vi "Day4_Statistics.vi"() -> ()   [LabVIEW 2025]
uses:
  <vilib>/Platform/TimedLoop/XDataNode/timing_clust.ctl
  <vilib>/Platform/TimedLoop/XDataNode/nitl_modes.ctl
  <vilib>/Platform/TimedLoop/XDataNode/wakeup.ctl
  <vilib>/Utility/error.llb/Trim Whitespace One-Sided.vi
  <vilib>/Instr/_visa.llb/VISA Configure Serial Port (Instr).vi
  <vilib>/platform/TimedLoop/XDataNode/XDataNode.xnode
  <vilib>/Platform/TimedLoop/XDataNode/XDNodeRunTimeDep.lvlib
  <vilib>/ptbypt/NI_PtbyPt.lvlib
panel:
  out "Max":dbl
  out "Min":dbl
  out "Mean":dbl
  out "Std Dev":dbl
  out "mean":dbl format="%0.2f"
  out "ADC (mv)":dbl
  out "Touch Pin":dbl
  out "Hall Sensor":dbl
  out "Timestamp":dbl
  in  "stop":bool
  # "Day 4: Statistics engine using a custom SubVI. Collects last 20 Touch Pin readings and computes live stats"
  # "Mean PtByPt: continuous running average since session start"
  # "Stats SubVI outputs: computed from a rolling buffer of the last 20 Touch Pin samples."
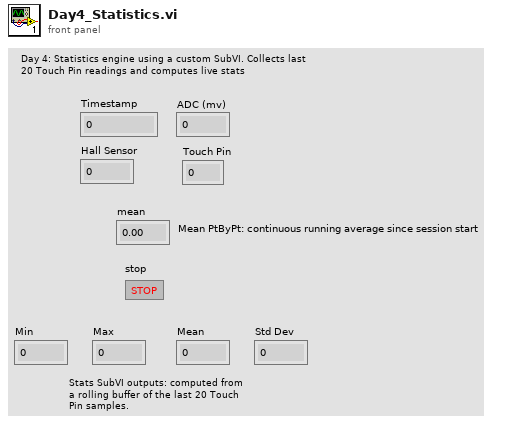
[diagram p1: front panel]
types:
  T1 = typedef "XDNodeRunTimeDep.lvlib/timing_clust.ctl" = cluster{"Expected End [f-1]":u64, "Actual End [f-1]":u64, "Finished Late? [f-1]":bool, "Expected End [i-1]":u64, "Actual End [i-1]":u64, "Finished Late? [i-1]":bool, "Expected Start [i]":u64, "Actual Start [i]":u64, "Expected Start [f]":u64, "Actual Start [f]":u64, "Source Name":string, "Structure Name":string, "Period":i64, "Deadline":i64, "Offset":i64, "Start":i64, "Priority":i32, "Timeout":i32, "Mode":T2, "Wakeup Reason":T3, "Error":errorcluster, "Source Type":string, "Secondary Source Type":string, "Global End Time":u64, "Global Start Time":u64, "Frame Duration":u64, "Iteration Duration":u64, "Assigned CPU":i32, "I/O Scan Engine Mode":u32}
  T2 = typedef "XDNodeRunTimeDep.lvlib/nitl_modes.ctl" = enum32{"No Change", "Process missed periods, maintain original phase", "Discard missed periods, maintain original phase", "Process missed periods, ignore original phase", "Discard missed periods, ignore original phase"}
  T3 = typedef "XDNodeRunTimeDep.lvlib/wakeup.ctl" = enum32{"Normal", "Aborted", "Asynchronous wakeup", "Timing source error", "Timed loop error", "Timeout"}
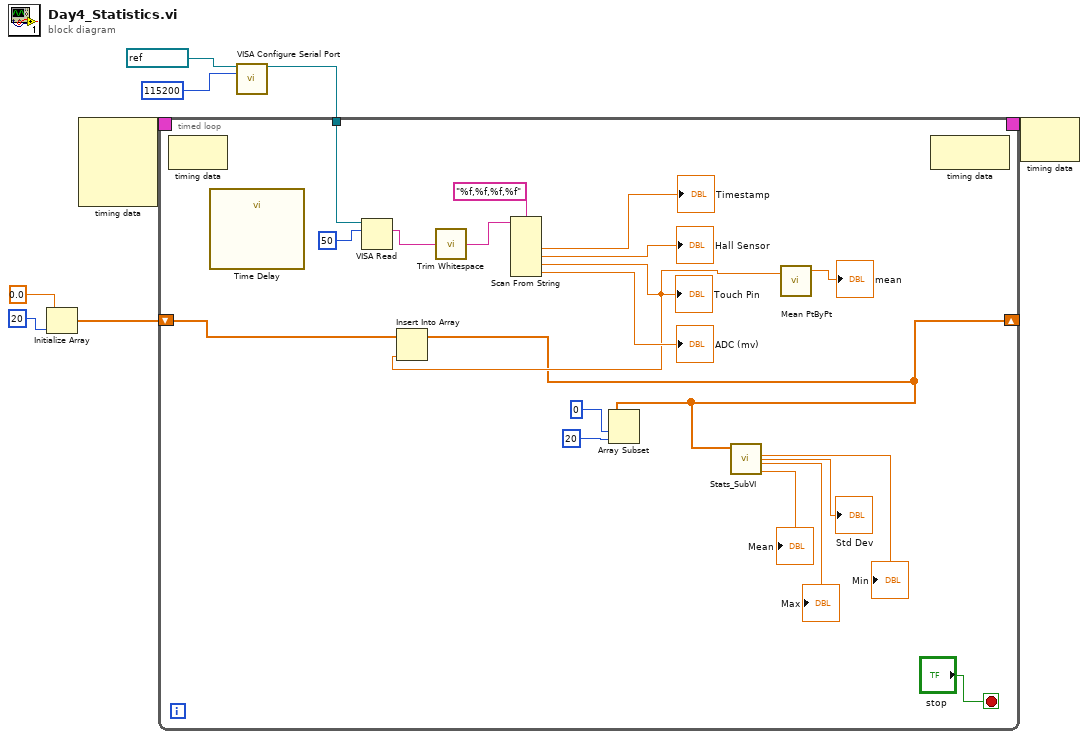
[diagram p0: block diagram]
diagram:
  n1 = Initialize Array "Initialize Array"(0.0 ("element"), 20 ("dimension size")) -> (w3:dbl[])
  n2 = node-c288() -> (w6:T1)  [unwired: 4 in]
  n3 = call-poly "VISA Configure Serial Port"("VISA resource name"=refnum<visa-resource-name> "COM3", "baud rate (9600)"=u32 115200) -> ("VISA resource name out"=w4:refnum<visa-resource-name>)  [unwired: 12 in, 1 out]
  n4 = timed-loop {
    timing: w6 -> [_]
    timing-out: [_] -> w5
    tunnel: w4 -> [w20]
    shift-right: [w13] -> _
    shift-left: w3 -> [w17]
    stop <- "stop" stop-if-true
    n5 = node-c288() -> ()  [unwired: 1 in, 1 out]
    n6 = call "Time Delay"() -> ()  [unwired: 11 in, 1 out]
    n7 = VISA Read(VISA resource name=w20, byte count=u32 50) -> (read buffer=w26:string)  [unwired: 1 in, 3 out]
    n8 = call <vilib>:"Trim Whitespace.vi"("string"=w26) -> ("trimmed string"=w25:string)  [unwired: 1 in]
    n9 = Scan From String "Scan From String"(format string="%f,%f,%f,%f", input string=w25) -> (output 1=→"Timestamp":dbl, output 2=→"Hall Sensor":dbl, output 3=w16:dbl, output 4=→"ADC (mv)":dbl)  [unwired: 6 in, 3 out]
    "Touch Pin" <- w16
    n10 = Insert Into Array "Insert Into Array"(array=w17, new element=w16) -> (w13:dbl[])  [unwired: 1 in]
    n11 = Array Subset "Array Subset"(array=w13, index=0, length=20) -> ()  [unwired: 1 out]
    n12 = call "Stats_SubVI.vi"("Input Array"=w13) -> ("Std Dev"=→"Std Dev":dbl, "Mean"=→"Mean":dbl, "Max"=→"Max":dbl, "Min"=→"Min":dbl)
    n13 = call <vilib>:"Mean PtByPt.vi"("x"=w16) -> ("mean"=→"mean":dbl)  [unwired: 3 in, 1 out]
    n14 = node-c288() -> ()  [unwired: 1 in, 1 out]
  }
  n15 = node-c288(w5) -> ()  [unwired: 1 out]
